vi "表格编辑.vi"(8 "新元素/子数组":string[](array[string]), 9 "活动单元格:单元格背景色":u32(colorbox), 11 "MCListbox引用句柄":refnum<vi>) -> ()   [LabVIEW 2013]
panel:
  out "表格总行数":u32=5
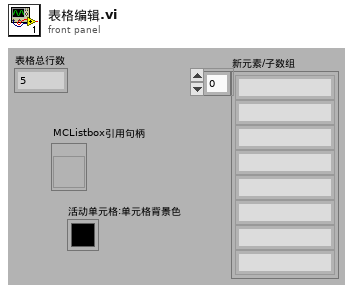
[diagram p1: front panel]
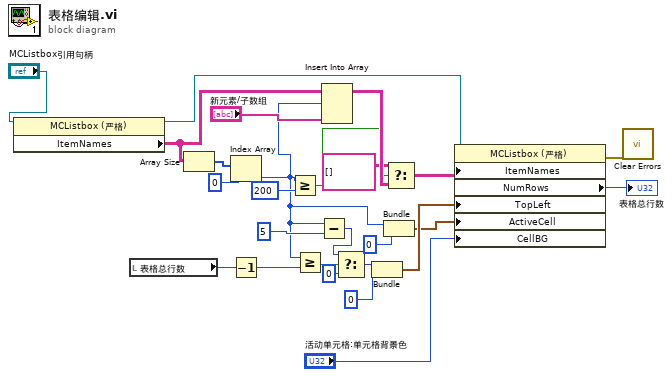
[diagram p0: block diagram]
diagram:
  n1 = property class="MCListbox (严格)"(reference="MCListbox引用句柄") -> (reference out=w23:refnum<vi>, "ItemNames"=w18:string[][])  [unwired: 1 in, 1 out]
  n2 = local read "表格总行数"() -> (w10:u32)
  n3 = Array Size(array=w18) -> (size(s)=w19:i32[])
  n4 = Index Array(array=w19, index=0 ("索引")) -> (element=w3:i32)
  n5 = Decrement(x=w10) -> (x-1=w9:u32)
  n6 = Greater Or Equal?(x=w3, y=200) -> (x >= y?=w15:bool)
  n7 = Greater Or Equal?(x=w3, y=w9) -> (x >= y?=w14:bool)
  n8 = Subtract(x=w3, y=5 ("保留行数")) -> (x-y=w11:i32)
  n9 = Insert Into Array(array=w18, index (row)=w3, new element="新元素/子数组") -> (w25:string[][])  [unwired: 1 in]
  n10 = Select(t=w11, s=w14, f=0) -> (s? t:f=w7:i32)
  n11 = Bundle("f"=w7, 0) -> (w8:cluster{"f":i32, i32})  [unwired: 1 out]
  n12 = Bundle(w3, 0) -> (w4:cluster{i32, i32})  [unwired: 1 out]
  n13 = Select(t=string[][] [], s=w15, f=w25) -> (s? t:f=w22:string[][])
  n14 = property class="MCListbox (严格)"(reference=w23, "ItemNames"=w22, "TopLeft"=w8, "ActiveCell"=w4, "CellBG"="活动单元格:单元格背景色") -> (error out=w1:errorcluster, "NumRows"=→"表格总行数":u32)  [unwired: 1 in, 1 out]
  n15 = call <vilib>:"Clear Errors.vi"("error in (no error)"=w1) -> ()  [unwired: 7 out]
